vi "ScanMonitor.PI.Multiple.Generate.vi"() -> ()   [LabVIEW 2019]
doc: "This example generates and starts multiple Programming Interface Scan Monitors.\n\n- Nanonis Programming Interface -"
uses:
  <vilib>/Utility/miscctls.llb/LVRectTypeDef.ctl
panel:
  in  "Generate.Number":i32=1 caption="Number of Scan Monitors to generate (1)"
  # "This example generates and starts multiple Programming Interface Scan Monitors.\n\nHow to use this vi:\n1) Choose the number of Scan Monitors to run\n2) Run the vi, the Scan Monitors will be generated and numbered in increasing order starting from 1"
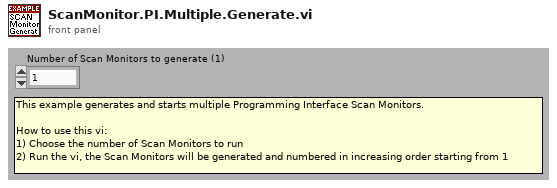
[diagram p1: front panel]
types:
  T1 = typedef "LVRectTypeDef.ctl" = cluster{"Left":i16, "Top":i16, "Right":i16, "Bottom":i16}
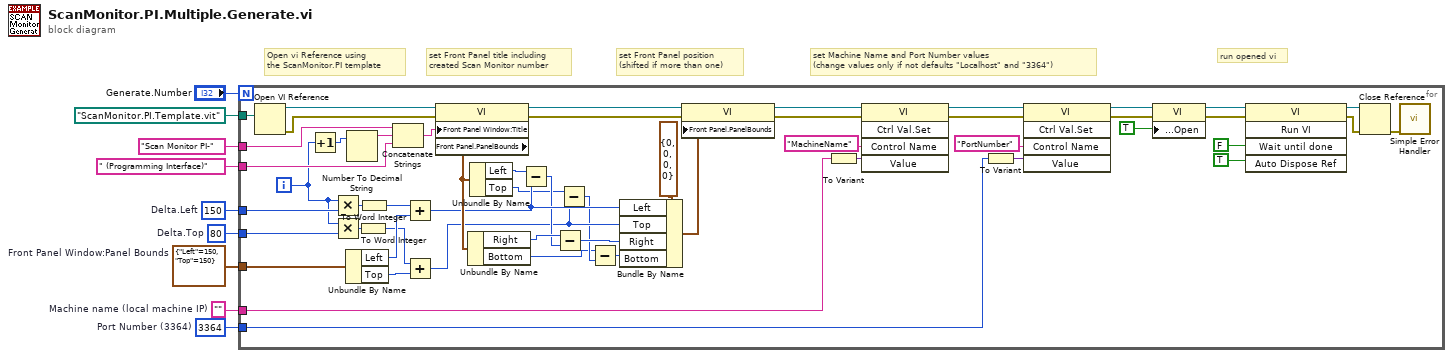
[diagram p0: block diagram]
diagram:
  w7 = u32 3364  # Port Number (3364)
  w1 = ""  # Machine name (local machine IP)
  w2 = 80  # Delta.Top
  w3 = 150  # Delta.Left
  w4 = cluster{"Left":i16, "Top":i16} {"Left"=150, "Top"=150}  # Front Panel Window:Panel Bounds
  # "set Machine Name and Port Number values\n(change values only if not defaults \"Localhost\" and \"3364\")"
  # "Open vi Reference using \nthe ScanMonitor.PI template"
  # "run opened vi"
  # "set Front Panel position\n(shifted if more than one)"
  # "set Front Panel title including \ncreated Scan Monitor number"
  n1 = for {
    N: "Generate.Number" -> [_]
    tunnel: path "ScanMonitor.PI.Template.vit" ("vi path") -> [w62]
    tunnel: w7 -> [w48]
    tunnel: "Scan Monitor PI-" ("Front Panel Window:Title") -> [w45]
    tunnel: " (Programming Interface)" ("Front Panel Window:Title") -> [w44]
    tunnel: w4 -> [w41]
    tunnel: w3 -> [w36]
    tunnel: w2 -> [w23]
    tunnel: w1 -> [w13]
    i -> [w20]
    n2 = Open VI Reference(vi path=w62) -> (vi reference=w50:refnum<vi>, error out=w49:errorcluster)  [unwired: 5 in]
    n3 = Increment(x=w20) -> (x+1=w43:i32)
    n4 = Multiply(x=w20, y=w36) -> (x*y=w22:i32)
    n5 = Multiply(x=w20, y=w23) -> (x*y=w21:i32)
    n6 = Unbundle By Name(w41) -> ("Left"=w37:i16, "Top"=w35:i16)
    n7 = Number To Decimal String(number=w43) -> (decimal integer string=w42:string)  [unwired: 1 in]
    n8 = To Word Integer(number=w21) -> (16bit integer=w18:i16)
    n9 = To Word Integer(number=w22) -> (16bit integer=w19:i16)
    n10 = Concatenate Strings(w45, w42, w44) -> (w46:string)
    n11 = Add(x=w19, y=w37) -> (x+y=w31:i16)
    n12 = Add(x=w18, y=w35) -> (x+y=w27:i16)
    n13 = property class="VI"(reference=w50, error in=w49, "Front Panel Window:Title"=w46) -> (reference out=w39:refnum<vi>, error out=w38:errorcluster, "Front Panel.PanelBounds"=w33:T1)
    n14 = Unbundle By Name(w33) -> ("Right"=w34:i16, "Bottom"=w25:i16)
    n15 = Unbundle By Name(w33) -> ("Left"=w32:i16, "Top"=w28:i16)
    n16 = Subtract(x=w32, y=w31) -> (x-y=w30:i16)
    n17 = Subtract(x=w34, y=w30) -> (x-y=w29:i16)
    n18 = Subtract(x=w28, y=w27) -> (x-y=w26:i16)
    n19 = Subtract(x=w25, y=w26) -> (x-y=w24:i16)
    n20 = Bundle By Name(cluster=T1 {"Left"=0, "Top"=0, "Right"=0, "Bottom"=0} ("Front Panel Window:Panel Bounds"), "Left"=w31, "Top"=w27, "Right"=w29, "Bottom"=w24) -> (w40:T1)
    n21 = property class="VI"(reference=w39, error in=w38, "Front Panel.PanelBounds"=w40) -> (reference out=w17:refnum<vi>, error out=w15:errorcluster)
    n22 = To Variant(anything=w13) -> (Variant=w10:variant)
    n23 = invoke class="VI" method="Ctrl Val.Set"(reference=w17, error in=w15, "Control Name"="MachineName", "Value"=w10) -> (reference out=w16:refnum<vi>, error out=w14:errorcluster)  [unwired: 1 in, 3 out]
    n24 = To Variant(anything=w48) -> (Variant=w47:variant)
    n25 = invoke class="VI" method="Ctrl Val.Set"(reference=w16, error in=w14, "Control Name"="PortNumber", "Value"=w47) -> (reference out=w55:refnum<vi>, error out=w54:errorcluster)  [unwired: 1 in, 3 out]
    n26 = property class="VI"(reference=w55, error in=w54, "Front Panel Window:Open"=TRUE) -> (reference out=w57:refnum<vi>, error out=w56:errorcluster)
    n27 = invoke class="VI" method="Run VI"(reference=w57, error in=w56, "Wait until done"=FALSE ("Wait Until Done"), "Auto Dispose Ref"=TRUE ("Auto Dispose Reference")) -> (reference out=w53:refnum<vi>, error out=w52:errorcluster)  [unwired: 1 in, 3 out]
    n28 = Close Reference(reference=w53, error in (no error)=w52) -> (error out=w61:errorcluster)
    n29 = call <vilib>:"Simple Error Handler.vi"("error in (no error)"=w61) -> ()  [unwired: 4 in, 5 out]
  }
